vi "Is Folder (Directory).vi"(1 "Input Path":path) -> (0 "Is Folder?":bool)   [LabVIEW 2016, in "Error Manager.lvlib" / "Settings.lvclass"]
uses:
  Settings.lvclass
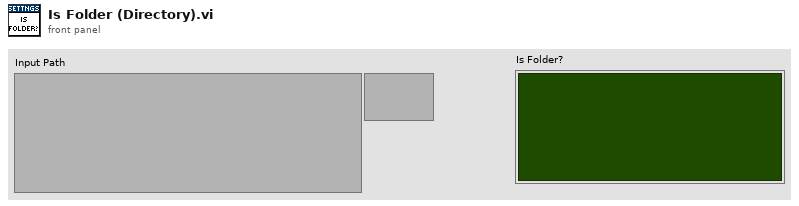
[diagram p1: front panel]
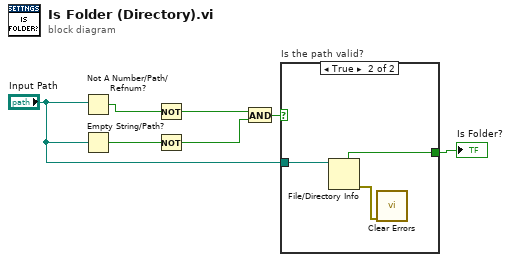
[diagram p0: block diagram]
diagram:
  n1 = Not A Number/Path/Refnum?(number/path/refnum="Input Path") -> (NaN/Path/Refnum?=w5:bool)
  n2 = Empty String/Path?(string/path="Input Path") -> (empty?=w6:bool)
  n3 = Not(x=w5) -> (.not. x?=w2:bool)
  n4 = Not(x=w6) -> (.not. x?=w1:bool)
  n5 = And(x=w2, y=w1) -> (x .and. y?=w3:bool)
  n6 = case "Is the path valid?" shown="True" w3 {
    tunnel: [_ w8] -> w7
    tunnel: "Input Path" -> [_ w10]
    frame False {
    }
    frame True {
      n7 = File/Directory Info(path=w10) -> (directory=w8:bool, error out=w9:errorcluster)  [unwired: 1 in, 5 out]
      n8 = call <vilib>:"Clear Errors.vi"("error in (no error)"=w9) -> ()  [unwired: 5 in, 2 out]
    }
  }
  "Is Folder?" <- w7
